vi "Read Config File.vi"(8 "error in (no error)":errorcluster, 11 "SM EOL Station Actor in":refnum<class "OPC Server.lvclass">) -> (0 "error out":errorcluster, 3 "SM EOL Station Actor out":refnum<class "OPC Server.lvclass">)   [LabVIEW 2021, in "OPC Server.lvlib" / "OPC Server.lvclass"]
uses:
  OPC Server.lvclass
  OPC Server.lvclass/OPC Server.ctl
  <vilib>/Utility/config.llb/Read Key (I32).vi
  <vilib>/Utility/config.llb/Read Key (String).vi
  <vilib>/Utility/config.llb/NI_LVConfig.lvlib
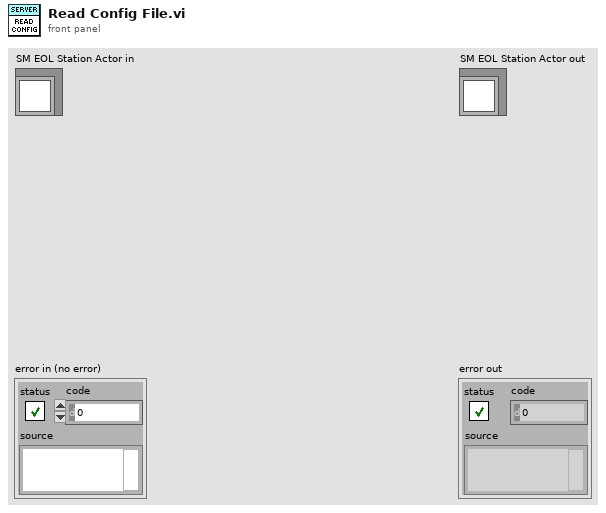
[diagram p1: front panel]
types:
  T1 = typedef "NI_LVConfig.lvlib/Config Data RefNum.ctl" = refnum<k1>
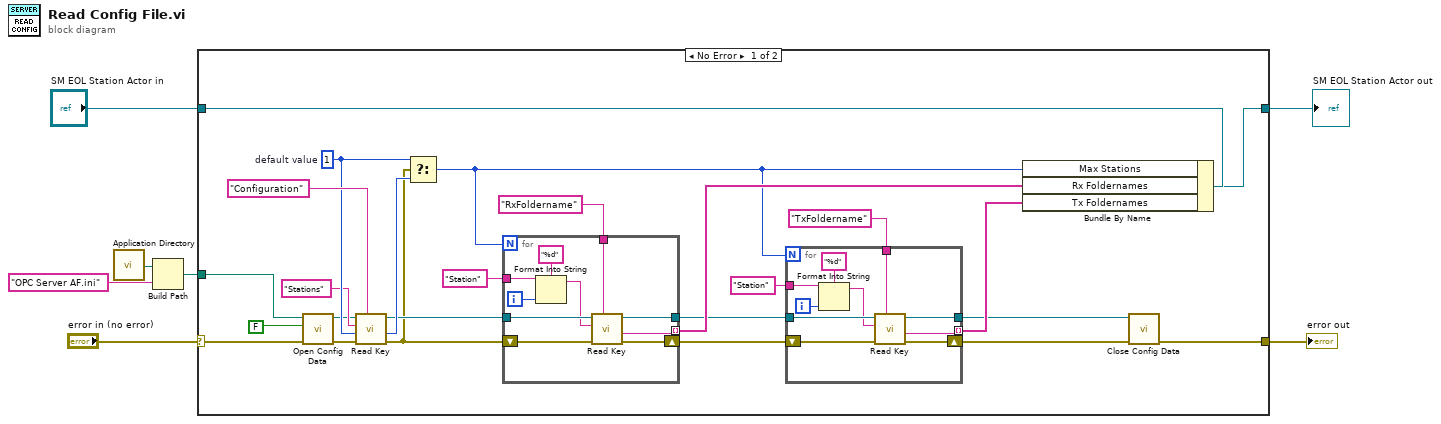
[diagram p0: block diagram]
diagram:
  n1 = call <vilib>:"Application Directory.vi"() -> ("Application Directory"=w3:path)
  n2 = Build Path(base path=w3, name or relative path="OPC Server AF.ini") -> (appended path=w1:path)
  n3 = case shown="No Error" "error in (no error)" {
    selector: "error in (no error)" -> [w19 w54]
    tunnel: [w18 w54] -> w6
    tunnel: [w24 w53] -> w4
    tunnel: "SM EOL Station Actor in" -> [w25 w53]
    tunnel: w1 -> [w20 _]
    frame No Error {
      w30 = 1  # default value
      n4 = call <vilib>:"Open Config Data.vi"("error in (no error)"=w19, "create file if necessary (T)"=FALSE, "configuration file path"=w20) -> ("error out"=w27:errorcluster, "refnum"=w28:T1)  [unwired: 6 in, 1 out]
      n5 = call-poly <vilib>:"Read Key.vi"("section"="Configuration", "error in (no error)"=w27, "default value"=w30, "key"="Stations", "refnum"=w28) -> ("error out"=w22:errorcluster, "value"=w31:i32, "refnum out"=w23:T1)  [unwired: 3 in, 1 out]
      n6 = Select(t=w30, s=w22, f=w31) -> (s? t:f=w15:i32)
      n7 = for {
        N: w15 -> [_]
        tunnel: [w50] -> w21 mode=indexing
        shift-right: [w49] -> w14
        shift-left: w22 -> [w51]
        tunnel: w23 -> [w52]
        tunnel: [w48] -> w11
        tunnel: "Station" ("key") -> [w47]
        tunnel: "RxFoldername" ("section") -> [w43]
        i -> [w45]
        n8 = Format Into String(format string="%d", initial string=w47, w45) -> (resulting string=w44:string)  [unwired: 1 in, 1 out]
        n9 = call-poly <vilib>:"Read Key.vi"("section"=w43, "error in (no error)"=w51, "key"=w44, "refnum"=w52) -> ("error out"=w49:errorcluster, "value"=w50:string, "refnum out"=w48:T1)  [unwired: 4 in, 1 out]
      }
      n10 = for {
        N: w15 -> [_]
        tunnel: [w40] -> w10 mode=indexing
        shift-right: [w39] -> w9
        shift-left: w14 -> [w41]
        tunnel: w11 -> [w42]
        tunnel: [w38] -> w8
        tunnel: "Station" ("key") -> [w37]
        tunnel: "TxFoldername" ("section") -> [w33]
        i -> [w35]
        n11 = Format Into String(format string="%d", initial string=w37, w35) -> (resulting string=w34:string)  [unwired: 1 in, 1 out]
        n12 = call-poly <vilib>:"Read Key.vi"("section"=w33, "error in (no error)"=w41, "key"=w34, "refnum"=w42) -> ("error out"=w39:errorcluster, "value"=w40:string, "refnum out"=w38:T1)  [unwired: 4 in, 1 out]
      }
      n13 = Bundle By Name(cluster=w25, "Max Stations"=w15, "Rx Foldernames"=w21, "Tx Foldernames"=w10) -> (w24:refnum<class "OPC Server.lvclass">)
      n14 = call <vilib>:"Close Config Data.vi"("error in (no error)"=w9, "refnum"=w8) -> ("error out"=w18:errorcluster)  [unwired: 8 in, 1 out]
    }
    frame Error {
    }
  }
  "error out" <- w6
  "SM EOL Station Actor out" <- w4
